vi "unflattenLengthFromXML_Scalar.vi"(8 "error in (no error)":errorcluster, 9 "lengthUnitInXML":T1, 10 "xmlString":string, 11 "lengthForType":dbl[unit]) -> (0 "error out":errorcluster, 3 "length":dbl[unit])   [LabVIEW 2016, in "UnitsAndXML.lvlib"]
uses:
  <userlib>/Common/UnitsAndXML/UnitsAndXML.lvlib
  <userlib>/Common/UnitsAndXML/FlattenItemWithUnitToXML/FlattenLengthToXML/LengthUnit.ctl
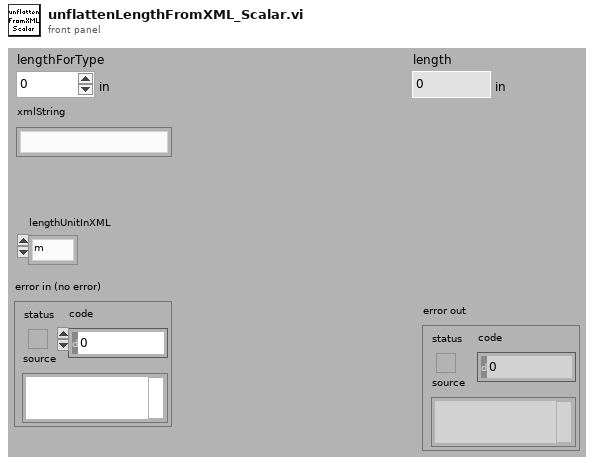
[diagram p1: front panel]
types:
  T1 = typedef "UnitsAndXML.lvlib/LengthUnit.ctl" = enum16{"m", "Angstrom", "AU", "chain", "cm", "cubit", "fathom", "fermi", "ft", "furlong", "hubble", "in", "ly", "mi", "mm", "rod", "um", "yd"}
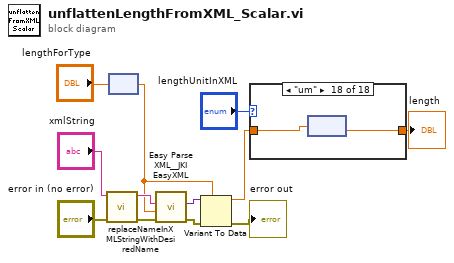
[diagram p0: block diagram]
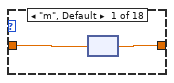
[diagram p2: hidden frame]
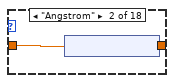
[diagram p3: hidden frame]
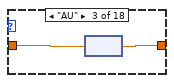
[diagram p4: hidden frame]
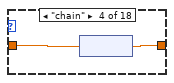
[diagram p5: hidden frame]
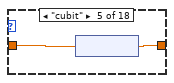
[diagram p6: hidden frame]
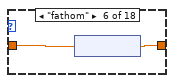
[diagram p7: hidden frame]
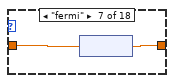
[diagram p8: hidden frame]
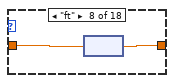
[diagram p9: hidden frame]
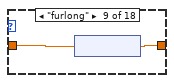
[diagram p10: hidden frame]
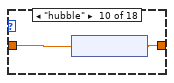
[diagram p11: hidden frame]
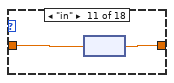
[diagram p12: hidden frame]
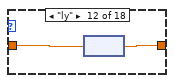
[diagram p13: hidden frame]
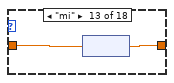
[diagram p14: hidden frame]
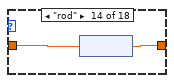
[diagram p15: hidden frame]
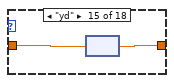
[diagram p16: hidden frame]
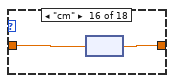
[diagram p17: hidden frame]
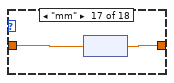
[diagram p18: hidden frame]
diagram:
  n1 = call <userlib>:"replaceNameInXMLStringWithDesiredName.vi"("error in"="error in (no error)", "xmlString"="xmlString") -> ("error out"=w4:errorcluster, "revisedXMLString"=w10:string)  [unwired: 8 in]
  n2 = node("lengthForType") -> (w8:dbl)
  n3 = call <vilib>:"Easy Parse XML__JKI EasyXML.vi"("error in (no error)"=w4, "LabVIEW Data (Type)"=w8, "XML String"=w10) -> ("error out"=w7:errorcluster, "LabVIEW Data"=w12:variant)  [unwired: 7 in]
  n4 = Variant To Data(error in=w7, type=w8, Variant=w12) -> (data=w2:dbl, error out=→"error out":errorcluster)
  n5 = case shown="\"um\"" "lengthUnitInXML" {
    tunnel: w2 -> [w14 w16 w18 w20 w21 w24 w26 w28 w30 w32 w34 w36 w38 w40 w42 w44 w46 w48]
    tunnel: [w13 w15 w17 w19 w22 w23 w25 w27 w29 w31 w33 w35 w37 w39 w41 w43 w45 w47] -> w1
    frame "m", Default {
      n6 = node(w14) -> (w13:dbl[unit])
    }
    frame "Angstrom" {
      n7 = node(w16) -> (w15:dbl[unit])
    }
    frame "AU" {
      n8 = node(w18) -> (w17:dbl[unit])
    }
    frame "chain" {
      n9 = node(w20) -> (w19:dbl[unit])
    }
    frame "cubit" {
      n10 = node(w21) -> (w22:dbl[unit])
    }
    frame "fathom" {
      n11 = node(w24) -> (w23:dbl[unit])
    }
    frame "fermi" {
      n12 = node(w26) -> (w25:dbl[unit])
    }
    frame "ft" {
      n13 = node(w28) -> (w27:dbl[unit])
    }
    frame "furlong" {
      n14 = node(w30) -> (w29:dbl[unit])
    }
    frame "hubble" {
      n15 = node(w32) -> (w31:dbl[unit])
    }
    frame "in" {
      n16 = node(w34) -> (w33:dbl[unit])
    }
    frame "ly" {
      n17 = node(w36) -> (w35:dbl[unit])
    }
    frame "mi" {
      n18 = node(w38) -> (w37:dbl[unit])
    }
    frame "rod" {
      n19 = node(w40) -> (w39:dbl[unit])
    }
    frame "yd" {
      n20 = node(w42) -> (w41:dbl[unit])
    }
    frame "cm" {
      n21 = node(w44) -> (w43:dbl[unit])
    }
    frame "mm" {
      n22 = node(w46) -> (w45:dbl[unit])
    }
    frame "um" {
      n23 = node(w48) -> (w47:dbl[unit])
    }
  }
  "length" <- w1
